vi "SS_FPGA_Drop1_all_in_v2.vi"() -> ()   [LabVIEW 2016]
uses:
  <vilib>/rvi/Emulation/niFpgaGetClockAttributes.vi
  <vilib>/rvi/Emulation/niFpgaSctlEmulationGetInTimedLoop.vi
  <vilib>/rvi/Emulation/niFpgaEmulationReportErrorSimple.vi
  <vilib>/rvi/Emulation/niFpgaCriticalErrorInLSC.vi
  <vilib>/rvi/Emulation/niFpgaProcessEmulError.vi
  <vilib>/rvi/eio/common/nirviEmuTemplateMethod_errors.vi
  <vilib>/eio/EIONode/EIONode.xnode
  <vilib>/rvi/FXPMathLib/FxpMul/XNode/nifxpmath_Multiplier.xnode
  <vilib>/rvi/FXPMathLib/FxpAdd/XNode/nifxpmath_Add.xnode
  <vilib>/rvi/FXPMathLib/sim/FxpSim.dll
panel:
  in  "Tab Control":T1(tab)
  in  "Start Acquisition":bool
  out "Actual Duration (ms)":u32
  out "Number of Loop 1 Samples":i32
  in  "Scan Rate (mSec) Loop 1":u32 caption="Count(mSec)"
  in  "Reset":bool
  in  "FSIS Interlock":bool
  out "x":bool
  out "Raw Data out Mod 1":fxp<+/-,24,-4>[](array[numeric])
  in  "offset mod 1":fxp<+/-,32,16>[](array[numeric])=[0.0, 0.0, 0.0, 0.0, 0.0, 0.0, 0.0, 0.0, 0.0, 0.0, 0.0, 0.0, 0.0, 0.0, 0.0, 0.0]
  in  "cal mod 1":fxp<+/-,32,16>[](array[numeric])=[10.0, 10.0, 10.0, 10.0, 10.0, 10.0, 10.0, 10.0, 10.0, 10.0, 10.0, 10.0, 10.0, 10.0, 10.0, 10.0]
  out "Cal value out Mod 1":sgl[](array[numeric])
  out "PTF - No Operations Mod 1":bool[](array[boolean])
  in  "lower limit \nNOOP mod 1":sgl[](array[numeric])=[0.0, 0.0, 0.0, 0.0, 0.0, 0.0, 0.0, 0.0, 0.0, 0.0, 0.0, 0.0, 0.0, 0.0, 0.0, 0.0]
  in  "upper limit \nOKOP mod 1":sgl[](array[numeric])=[0.0, 0.0, 0.0, 0.0, 0.0, 0.0, 0.0, 0.0, 0.0, 0.0, 0.0, 0.0, 0.0, 0.0, 0.0, 0.0]
  out "PTF - Warning Mod 1":bool[](array[boolean])
  in  "NOOPS Fault Filter mod 1":u16[](array[numeric])=[0, 0, 0, 0, 0, 0, 0, 0, 0, 0, 0, 0, 0, 0, 0, 0]
  out "Raw Data out Mod 2":fxp<+/-,24,-4>[](array[numeric]) format="%.27g"
  in  "offset mod 2":fxp<+/-,32,16>[](array[numeric])=[0.0, 0.0, 0.0, 0.0, 0.0, 0.0, 0.0, 0.0, 0.0, 0.0, 0.0, 0.0, 0.0, 0.0, 0.0, 0.0]
  in  "cal mod 2":fxp<+/-,32,16>[](array[numeric])=[0.0, 0.0, 0.0, 0.0, 0.0, 0.0, 0.0, 0.0, 0.0, 0.0, 0.0, 0.0, 0.0, 0.0, 0.0, 0.0]
  out "PTF - No Operations Mod 2":bool[](array[boolean])
  in  "lower limit \nNOOP mod 2":sgl[](array[numeric])=[0.0, 0.0, 0.0, 0.0, 0.0, 0.0, 0.0, 0.0, 0.0, 0.0, 0.0, 0.0, 0.0, 0.0, 0.0, 0.0]
  in  "upper limit \nOKOP mod 2":sgl[](array[numeric])=[0.0, 0.0, 0.0, 0.0, 0.0, 0.0, 0.0, 0.0, 0.0, 0.0, 0.0, 0.0, 0.0, 0.0, 0.0, 0.0]
  out "Cal value out Mod 2":sgl[](array[numeric])
  out "PTF - Warning Mod 2":bool[](array[boolean])
  in  "NOOPS Fault Filter mod 2":u16[](array[numeric])=[0, 0, 0, 0, 0, 0, 0, 0, 0, 0, 0, 0, 0, 0, 0, 0]
  out "Raw Data out Mod 3":fxp<+/-,24,-4>[](array[numeric]) format="%.27g"
  in  "cal mod 3":fxp<+/-,32,16>[](array[numeric])=[0.0, 0.0, 0.0, 0.0, 0.0, 0.0, 0.0, 0.0, 0.0, 0.0, 0.0, 0.0, 0.0, 0.0, 0.0, 0.0]
  in  "offset mod 3":fxp<+/-,32,16>[](array[numeric])=[0.0, 0.0, 0.0, 0.0, 0.0, 0.0, 0.0, 0.0, 0.0, 0.0, 0.0, 0.0, 0.0, 0.0, 0.0, 0.0]
  out "PTF - No Operations Mod 3":bool[](array[boolean])
  in  "lower limit\nNOOP mod 3":sgl[](array[numeric])=[0.0, 0.0, 0.0, 0.0, 0.0, 0.0, 0.0, 0.0, 0.0, 0.0, 0.0, 0.0, 0.0, 0.0, 0.0, 0.0]
  in  "upper limit\nOKOP mod 3":sgl[](array[numeric])=[0.0, 0.0, 0.0, 0.0, 0.0, 0.0, 0.0, 0.0, 0.0, 0.0, 0.0, 0.0, 0.0, 0.0, 0.0, 0.0]
  out "PTF - Warning Mod 3":bool[](array[boolean])
  out "Cal value out Mod 3":sgl[](array[numeric])
  in  "NOOPS Fault Filter mod 3":u16[](array[numeric])=[0, 0, 0, 0, 0, 0, 0, 0, 0, 0, 0, 0, 0, 0, 0, 0]
  # "CHANNEL ID"
  # "1"
  # "SS Source Body Flow\n\nSS Source Body Temperature\n\nSS Grid 1 Flow\n\nSS Grid 1 Temperature\n\nSS Grid 2 Flow\n\nSS Grid 2 Temperature\n\nSS Grid 3 Flow\n\nSS Grid 3 Temperature\n\nSS Grid 4/1st Stage Neutraliser Flow\n\nSS Grid 4/1st Stage Neutraliser Temperature\n\nSS 2nd Stage Neutraliser Flow\n\nSS 2nd Stage Neutraliser Temperature\n\nSS PINI Backplate Flow\n\nSS PINI Backplate Temperature\n\nSS Duct Scraper Flow\n\nSS Duct Scraper Temperature"
  # "2"
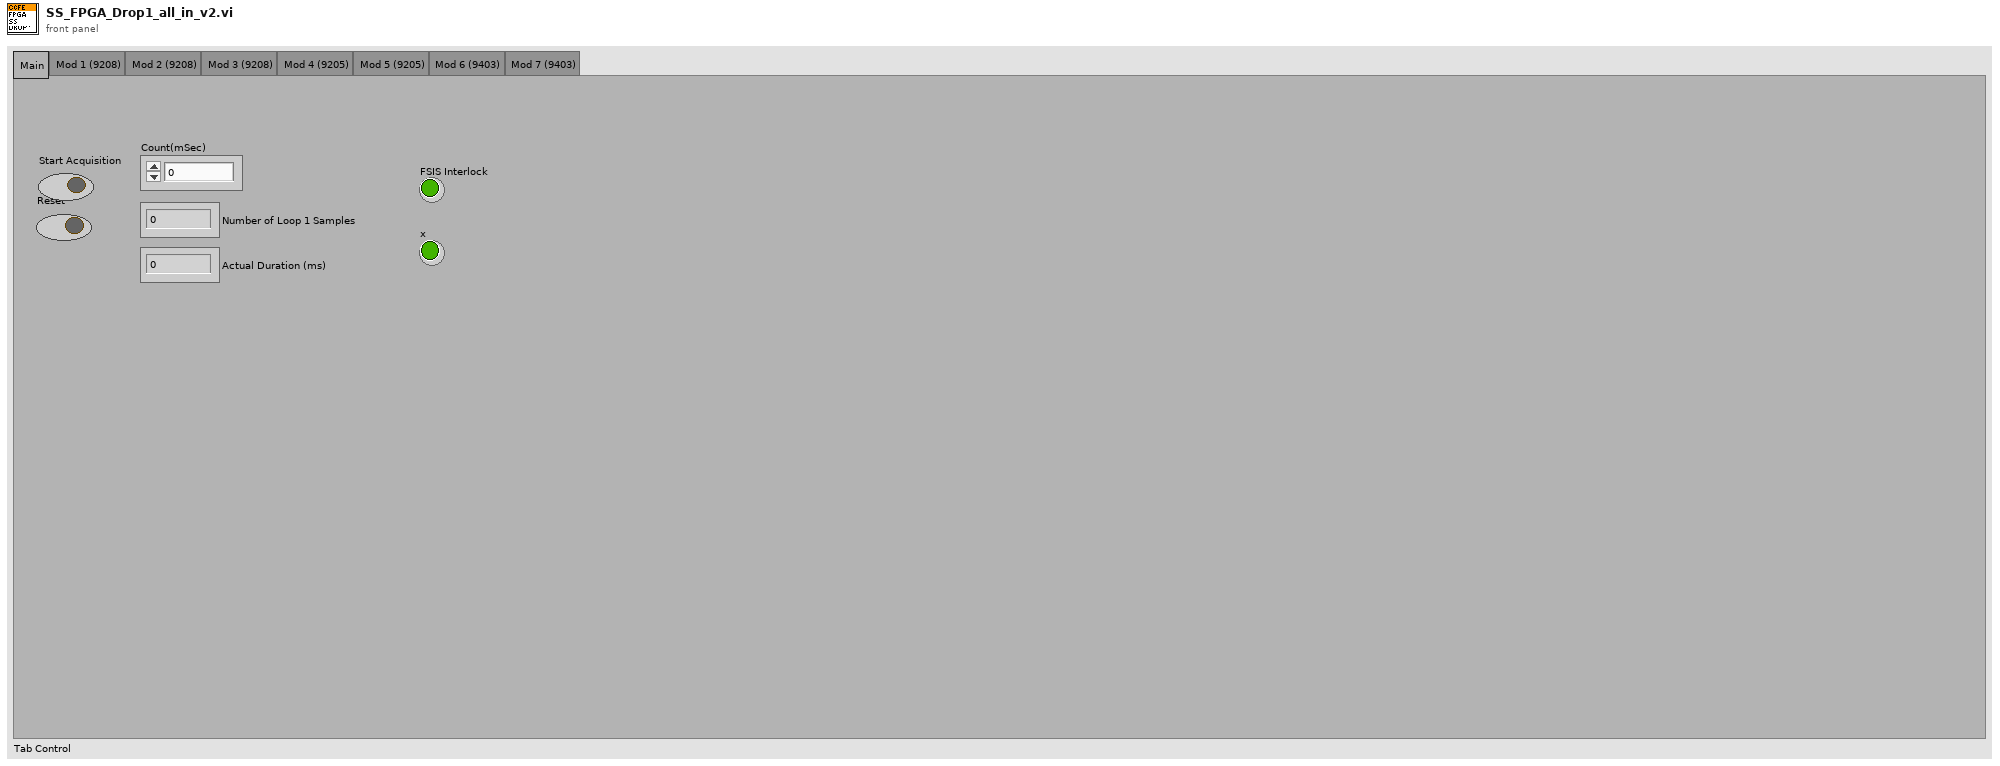
[diagram p1: front panel]
types:
  T1 = enum32{"Main", "Mod 1 (9208)", "Mod 2 (9208)", "Mod 3 (9208)", "Mod 4 (9205)", "Mod 5 (9205)", "Mod 6 (9403)", "Mod 7 (9403)"}
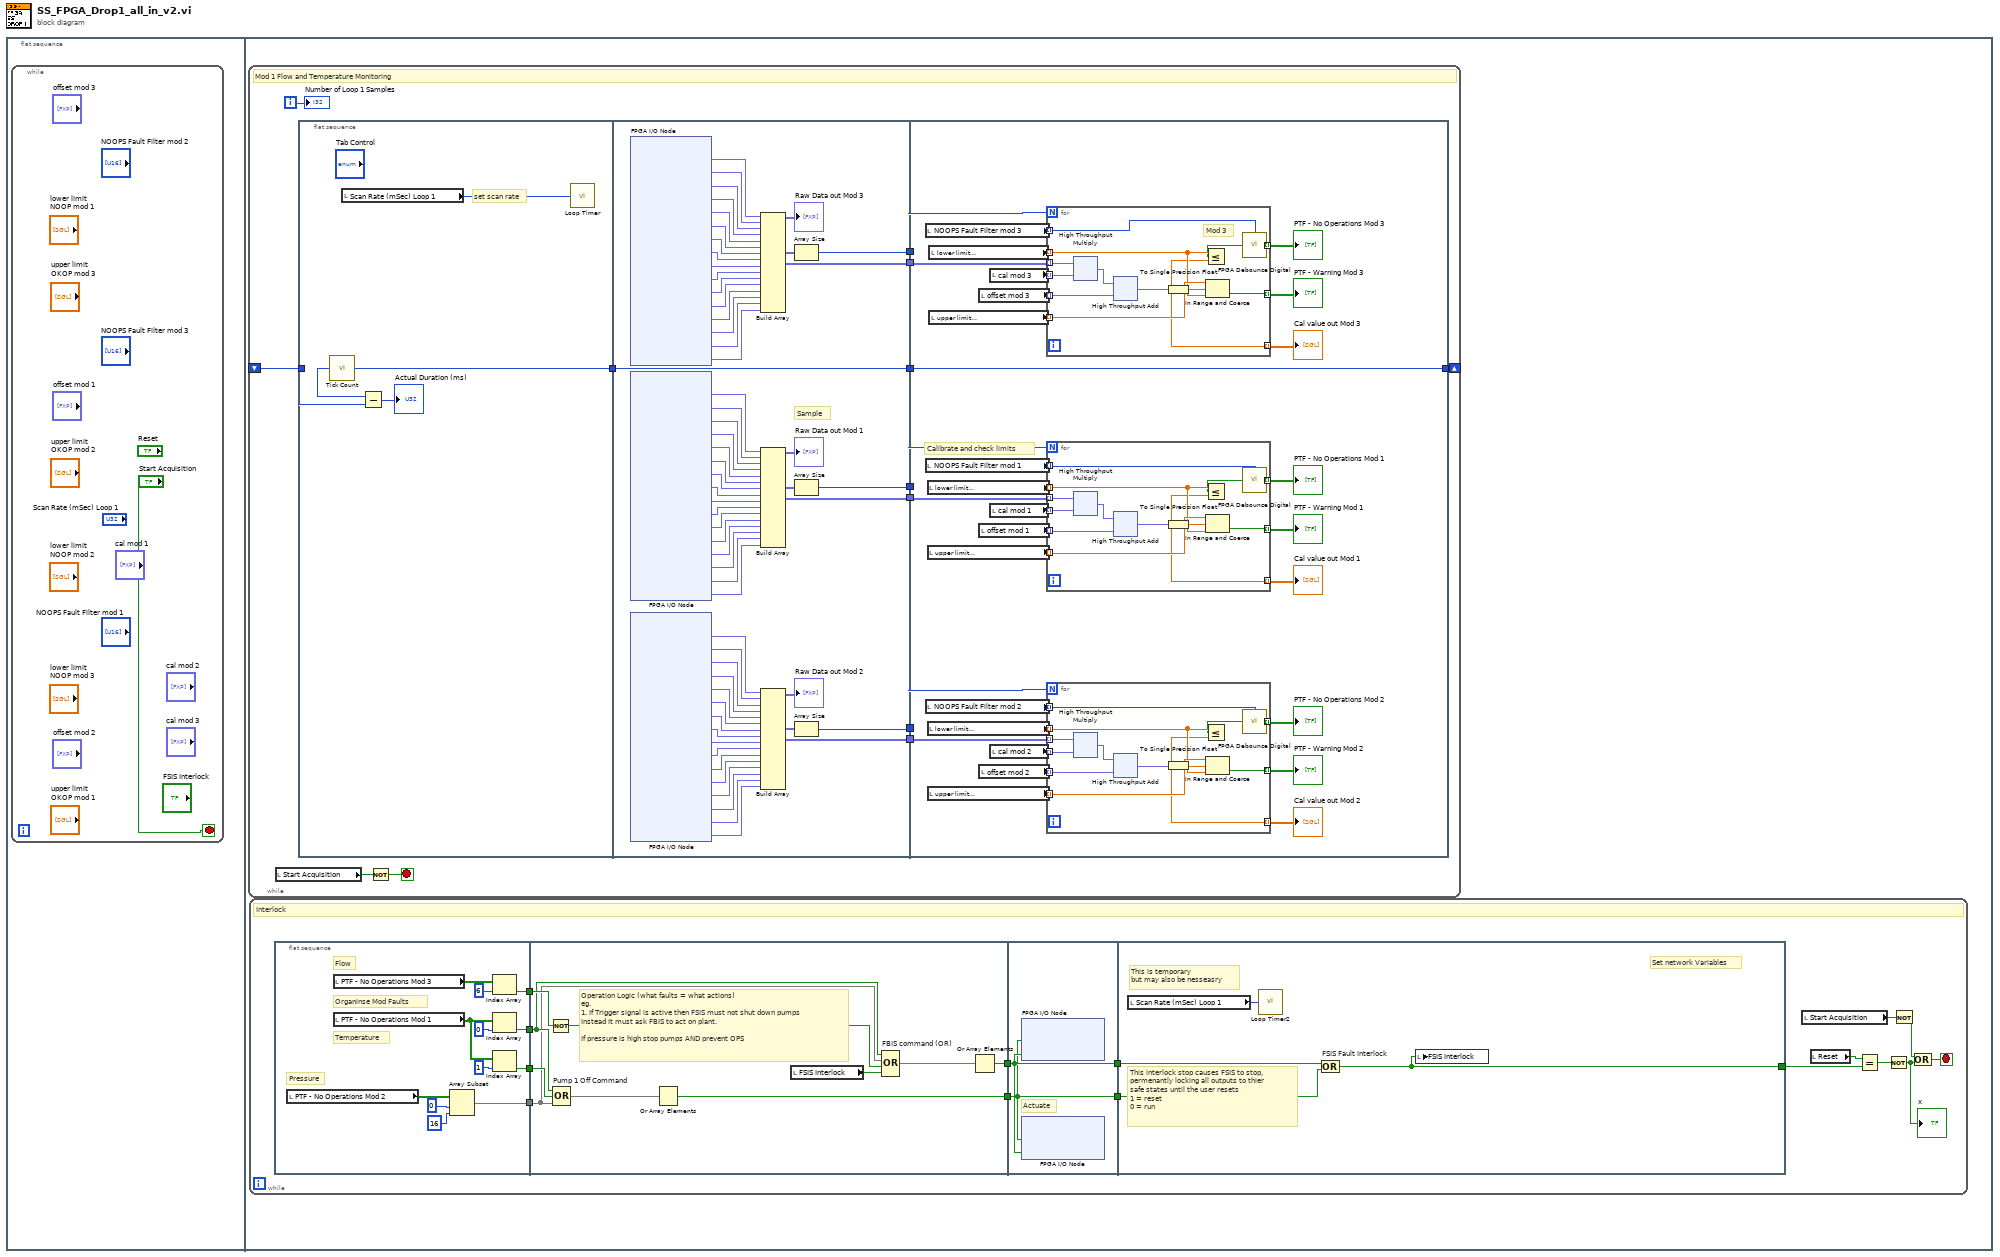
[diagram p0: block diagram]
diagram:
  n1 = flat-sequence {
    frame #0 {
      n2 = while {
        stop <- "Start Acquisition" stop-if-true
      }
    }
    frame #1 {
      n3 = while {
        shift-right: [w56] -> _
        shift-left: _ -> [w54]
        i -> [w57]
        stop <- w53 stop-if-true
        # "Mod 1 Flow and Temperature Monitoring"
        n4 = local read "Start Acquisition"() -> (w52:bool)
        n5 = flat-sequence {
          tunnel: [w58] -> w55
          tunnel: w54 -> [w59]
          tunnel: w55 -> [w100]
          tunnel: [w100] -> w51
          tunnel: [w70] -> w50
          tunnel: [w66] -> w49
          tunnel: [w65] -> w48
          tunnel: [w63] -> w47
          tunnel: [w64] -> w46
          tunnel: [w62] -> w45
          tunnel: w51 -> [w147]
          tunnel: w50 -> [w136]
          tunnel: w49 -> [w135]
          tunnel: w48 -> [w146]
          tunnel: w47 -> [w141]
          tunnel: w46 -> [w134]
          tunnel: w45 -> [w133]
          tunnel: [w147] -> w56
          frame #0 {
            # "set scan rate"
            n6 = call "Tick Count"() -> ("Tick Count(mSec)"=w58:u32)
            n7 = local read "Scan Rate (mSec) Loop 1"() -> (w61:u32)
            n8 = Subtract(x=w58, y=w59) -> (x-y=→"Actual Duration (ms)":u32)
            n9 = call "Loop Timer"("Count(mSec)"=w61) -> ()  [unwired: 1 out]
          }
          frame #1 {
            # "Sample"
            n10 = xnode "FPGA I/O Node"() -> ("Mod3/AI0"=w99:fxp<+/-,24,-4>, "Mod3/AI1"=w98:fxp<+/-,24,-4>, "Mod3/AI2"=w97:fxp<+/-,24,-4>, "Mod3/AI3"=w96:fxp<+/-,24,-4>, "Mod3/AI4"=w95:fxp<+/-,24,-4>, "Mod3/AI5"=w94:fxp<+/-,24,-4>, "Mod3/AI6"=w93:fxp<+/-,24,-4>, "Mod3/AI7"=w92:fxp<+/-,24,-4>, "Mod3/AI8"=w91:fxp<+/-,24,-4>, "Mod3/AI9"=w90:fxp<+/-,24,-4>, "Mod3/AI10"=w89:fxp<+/-,24,-4>, "Mod3/AI11"=w88:fxp<+/-,24,-4>, "Mod3/AI12"=w87:fxp<+/-,24,-4>, "Mod3/AI13"=w69:fxp<+/-,24,-4>, "Mod3/AI14"=w68:fxp<+/-,24,-4>, "Mod3/AI15"=w67:fxp<+/-,24,-4>)  [unwired: 16 in, 16 out]
            n11 = xnode "FPGA I/O Node"() -> ("Mod1/AI0"=w116:fxp<+/-,24,-4>, "Mod1/AI1"=w115:fxp<+/-,24,-4>, "Mod1/AI2"=w114:fxp<+/-,24,-4>, "Mod1/AI3"=w113:fxp<+/-,24,-4>, "Mod1/AI4"=w112:fxp<+/-,24,-4>, "Mod1/AI5"=w111:fxp<+/-,24,-4>, "Mod1/AI6"=w110:fxp<+/-,24,-4>, "Mod1/AI7"=w109:fxp<+/-,24,-4>, "Mod1/AI8"=w108:fxp<+/-,24,-4>, "Mod1/AI9"=w107:fxp<+/-,24,-4>, "Mod1/AI10"=w106:fxp<+/-,24,-4>, "Mod1/AI11"=w105:fxp<+/-,24,-4>, "Mod1/AI12"=w104:fxp<+/-,24,-4>, "Mod1/AI13"=w103:fxp<+/-,24,-4>, "Mod1/AI14"=w102:fxp<+/-,24,-4>, "Mod1/AI15"=w101:fxp<+/-,24,-4>)  [unwired: 16 in, 16 out]
            n12 = xnode "FPGA I/O Node"() -> ("Mod2/AI0"=w71:fxp<+/-,24,-4>, "Mod2/AI1"=w72:fxp<+/-,24,-4>, "Mod2/AI2"=w73:fxp<+/-,24,-4>, "Mod2/AI3"=w74:fxp<+/-,24,-4>, "Mod2/AI4"=w75:fxp<+/-,24,-4>, "Mod2/AI5"=w76:fxp<+/-,24,-4>, "Mod2/AI6"=w77:fxp<+/-,24,-4>, "Mod2/AI7"=w78:fxp<+/-,24,-4>, "Mod2/AI8"=w79:fxp<+/-,24,-4>, "Mod2/AI9"=w80:fxp<+/-,24,-4>, "Mod2/AI10"=w81:fxp<+/-,24,-4>, "Mod2/AI11"=w82:fxp<+/-,24,-4>, "Mod2/AI12"=w83:fxp<+/-,24,-4>, "Mod2/AI13"=w84:fxp<+/-,24,-4>, "Mod2/AI14"=w85:fxp<+/-,24,-4>, "Mod2/AI15"=w86:fxp<+/-,24,-4>)  [unwired: 16 in, 16 out]
            n13 = Build Array(w99, w98, w97, w96, w95, w94, w93, w92, w91, w90, w89, w88, w87, w69, w68, w67) -> (w63:fxp<+/-,24,-4>[])
            "Raw Data out Mod 3" <- w63
            n14 = Build Array(w116, w115, w114, w113, w112, w111, w110, w109, w108, w107, w106, w105, w104, w103, w102, w101) -> (w66:fxp<+/-,24,-4>[])
            "Raw Data out Mod 1" <- w66
            n15 = Build Array(w71, w72, w73, w74, w75, w76, w77, w78, w79, w80, w81, w82, w83, w84, w85, w86) -> (w65:fxp<+/-,24,-4>[])
            "Raw Data out Mod 2" <- w65
            n16 = Array Size(array=w63) -> (size(s)=w62:i32)
            n17 = Array Size(array=w66) -> (size(s)=w70:i32)
            n18 = Array Size(array=w65) -> (size(s)=w64:i32)
          }
          frame #2 {
            # "Calibrate and check limits"
            n19 = local read "NOOPS Fault Filter mod 3"() -> (w119:u16[])
            n20 = local read "NOOPS Fault Filter mod 1"() -> (w120:u16[])
            n21 = local read "NOOPS Fault Filter mod 2"() -> (w118:u16[])
            n22 = local read "lower limit \nNOOP mod 1"() -> (w132:sgl[])
            n23 = local read "upper limit \nOKOP mod 1"() -> (w131:sgl[])
            n24 = local read "lower limit \nNOOP mod 2"() -> (w142:sgl[])
            n25 = local read "upper limit \nOKOP mod 2"() -> (w143:sgl[])
            n26 = local read "lower limit\nNOOP mod 3"() -> (w138:sgl[])
            n27 = local read "upper limit\nOKOP mod 3"() -> (w137:sgl[])
            n28 = local read "offset mod 3"() -> (w139:fxp<+/-,32,16>[])
            n29 = local read "offset mod 1"() -> (w129:fxp<+/-,32,16>[])
            n30 = local read "offset mod 2"() -> (w145:fxp<+/-,32,16>[])
            n31 = local read "cal mod 3"() -> (w140:fxp<+/-,32,16>[])
            n32 = local read "cal mod 1"() -> (w130:fxp<+/-,32,16>[])
            n33 = local read "cal mod 2"() -> (w144:fxp<+/-,32,16>[])
            n34 = for {
              N: w133 -> [_]
              tunnel: w140 -> [w164] mode=indexing
              tunnel: w139 -> [w163] mode=indexing
              tunnel: w141 -> [w165] mode=indexing
              tunnel: [w160] -> w128 mode=indexing
              tunnel: w137 -> [w170] mode=indexing
              tunnel: w138 -> [w169] mode=indexing
              tunnel: [w171] -> w126 mode=indexing
              tunnel: [w167] -> w125 mode=indexing
              tunnel: w119 -> [w166] mode=indexing
              # "Mod 3"
              n35 = xnode ("High Throughput Multiply")("x"=w165, "y"=w164) -> ("x*y"=w162:fxp<+/-,56,12>)
              n36 = xnode ("High Throughput Add")("x"=w162, "y"=w163) -> ("x+y"=w161:fxp<+/-,61,17>)
              n37 = To Single Precision Float(number=w161) -> (single precision float=w160:sgl)
              n38 = Less Or Equal?(x=w169, y=w160) -> (x <= y?=w168:bool)
              n39 = In Range and Coerce(upper limit=w170, x=w160, lower limit=w169) -> (In Range?=w171:bool)  [unwired: 1 out]
              n40 = call "FPGA Debounce Digital.vi"("Input Signal"=w168, "Cycles to Filter"=w166) -> ("Output Filtered Signal"=w167:bool)
            }
            "Cal value out Mod 3" <- w128
            "PTF - No Operations Mod 3" <- w125
            "PTF - Warning Mod 3" <- w126
            n41 = for {
              N: w136 -> [_]
              tunnel: w130 -> [w150] mode=indexing
              tunnel: w129 -> [w149] mode=indexing
              tunnel: w135 -> [w148] mode=indexing
              tunnel: w131 -> [w159] mode=indexing
              tunnel: w132 -> [w158] mode=indexing
              tunnel: [w156] -> w124 mode=indexing
              tunnel: [w155] -> w123 mode=indexing
              tunnel: w120 -> [w154] mode=indexing
              tunnel: [w151] -> w117 mode=indexing
              n42 = xnode ("High Throughput Multiply")("x"=w148, "y"=w150) -> ("x*y"=w152:fxp<+/-,56,12>)
              n43 = xnode ("High Throughput Add")("x"=w152, "y"=w149) -> ("x+y"=w153:fxp<+/-,61,17>)
              n44 = To Single Precision Float(number=w153) -> (single precision float=w151:sgl)
              n45 = Less Or Equal?(x=w158, y=w151) -> (x <= y?=w157:bool)
              n46 = In Range and Coerce(upper limit=w159, x=w151, lower limit=w158) -> (In Range?=w155:bool)  [unwired: 1 out]
              n47 = call "FPGA Debounce Digital.vi"("Input Signal"=w157, "Cycles to Filter"=w154) -> ("Output Filtered Signal"=w156:bool)
            }
            "Cal value out Mod 1" <- w117
            "PTF - No Operations Mod 1" <- w124
            "PTF - Warning Mod 1" <- w123
            n48 = for {
              N: w134 -> [_]
              tunnel: w144 -> [w177] mode=indexing
              tunnel: w145 -> [w175] mode=indexing
              tunnel: w146 -> [w176] mode=indexing
              tunnel: [w172] -> w127 mode=indexing
              tunnel: w143 -> [w182] mode=indexing
              tunnel: w142 -> [w181] mode=indexing
              tunnel: [w183] -> w121 mode=indexing
              tunnel: [w179] -> w122 mode=indexing
              tunnel: w118 -> [w178] mode=indexing
              n49 = xnode ("High Throughput Multiply")("x"=w176, "y"=w177) -> ("x*y"=w174:fxp<+/-,56,12>)
              n50 = xnode ("High Throughput Add")("x"=w174, "y"=w175) -> ("x+y"=w173:fxp<+/-,61,17>)
              n51 = To Single Precision Float(number=w173) -> (single precision float=w172:sgl)
              n52 = Less Or Equal?(x=w181, y=w172) -> (x <= y?=w180:bool)
              n53 = In Range and Coerce(upper limit=w182, x=w172, lower limit=w181) -> (In Range?=w183:bool)  [unwired: 1 out]
              n54 = call "FPGA Debounce Digital.vi"("Input Signal"=w180, "Cycles to Filter"=w178) -> ("Output Filtered Signal"=w179:bool)
            }
            "Cal value out Mod 2" <- w127
            "PTF - No Operations Mod 2" <- w122
            "PTF - Warning Mod 2" <- w121
          }
        }
        n55 = Not(x=w52) -> (.not. x?=w53:bool)
        "Number of Loop 1 Samples" <- w57
      }
      n56 = while {
        stop <- w7 stop-if-true
        # "Interlock"
        n57 = flat-sequence {
          tunnel: [w27] -> w15
          tunnel: [w24] -> w13
          tunnel: [w20] -> w12
          tunnel: [w17] -> w11
          tunnel: w15 -> [w36]
          tunnel: [w31] -> w14
          tunnel: w13 -> [w34]
          tunnel: w12 -> [w37]
          tunnel: w11 -> [w35]
          tunnel: [w32] -> w10
          tunnel: w14 -> [w40]
          tunnel: w10 -> [w39]
          tunnel: [w40] -> w9
          tunnel: [w39] -> w8
          tunnel: w9 -> [w43]
          tunnel: w8 -> [w42]
          tunnel: [w41] -> w5
          frame #0 {
            # "Flow"
            # "Temperature"
            # "Pressure"
            # "Organinse Mod Faults"
            n58 = local read "PTF - No Operations Mod 2"() -> (w23:bool[])
            n59 = local read "PTF - No Operations Mod 3"() -> (w21:bool[])
            n60 = local read "PTF - No Operations Mod 1"() -> (w18:bool[])
            n61 = Array Subset(array=w23, index=0, length=16 ("index")) -> (w24:bool[])
            n62 = Index Array(array=w21, index=6) -> (element=w20:bool)
            n63 = Index Array(array=w18, index=0) -> (element=w27:bool)
            n64 = Index Array(array=w18, index=1) -> (element=w17:bool)
          }
          frame #1 {
            # "Operation Logic (what faults = what actions)\neg.\n1. If Trigger signal is active then FSIS must not shut down pumps\nInstead It must ask FBIS to act on plant.\n\nIf pressure is high stop pumps AND prevent OPS"
            n65 = Not(x=w37) -> (.not. x?=w38:bool)
            n66 = Compound Arithmetic op=OR "Pump 1 Off Command"(w36, w35, w34) -> (w33:bool[])
            n67 = Or Array Elements(Boolean array=w33) -> (logical OR=w32:bool)
            n68 = local read "FSIS Interlock"() -> (w29:bool)
            n69 = Compound Arithmetic op=OR "FBIS command (OR)"(w36, w34, w38, w29) -> (w30:bool[])
            n70 = Or Array Elements(Boolean array=w30) -> (logical OR=w31:bool)
          }
          frame #2 {
            # "Actuate"
            n71 = xnode "FPGA I/O Node"("Mod7/DIO0"=w39, "Mod7/DIO1"=w40) -> ()  [unwired: 2 in, 2 out]
            n72 = xnode "FPGA I/O Node"("Mod6/DIO0"=w39, "Mod6/DIO1"=w40) -> ()  [unwired: 2 in, 2 out]
          }
          frame #3 {
            # "This interlock stop causes FSIS to stop,\npermenantly locking all outputs to thier \nsafe states until the user resets\n1 = reset\n0 = run"
            # "This is temporary\nbut may also be nesseasry"
            # "Set network Variables"
            n73 = local read "Scan Rate (mSec) Loop 1"() -> (w44:u32)
            n74 = call "Loop Timer2"("Count(mSec)"=w44) -> ()  [unwired: 1 out]
            n75 = Compound Arithmetic op=OR "FSIS Fault Interlock"(w43, w42) -> (w41:bool)
            n76 = local write "FSIS Interlock"(w41) -> ()
          }
        }
        n77 = local read "Start Acquisition"() -> (w16:bool)
        n78 = local read "Reset"() -> (w4:bool)
        n79 = Equal?(x=w4, y=w5) -> (x = y?=w3:bool)
        n80 = Not(x=w3) -> (.not. x?=w2:bool)
        "x" <- w2
        n81 = Not(x=w16) -> (.not. x?=w6:bool)
        n82 = Or(x=w6, y=w2) -> (x .or. y?=w7:bool)
      }
    }
  }
